vi "CIS.vi"(2 "Run uninterrupted?":bool, 3 "Device Category IN:":string(combo)="ATLAS18SS" caption="Device Category:", 4 "Batch No. IN:":string caption="Batch No.:", 5 "Wafer No. IN:":string caption="Wafer No.:", 6 "DB Serial No. IN:":string caption="DB Serial No.:") -> (0 "Done!":bool)   [LabVIEW 2018]
doc: "Performs Cis measurements according to ATLAS ITk Quality Control Specifications."
uses:
  InstrControl/Switching/Switching.lvclass
  general_VIs/globals/QC_MeasurementSetup.vi
  general_VIs/globals/QC_RunInformation.vi
  InstrControl/InstrumentSetup.vi
  InstrControl/SupplyControl/SupplyControl.lvclass
  InstrControl/LCRControl/LCRControl.lvclass
  InstrControl/ArduinoControl/ArduinoControl.lvclass
  <vilib>/Analysis/NI_AALBase.lvlib
  InstrControl/InstrControl.lvclass
panel:
  out "Tab Control 2":enum32{"Cis Setup", "Cis Scan"}(tab)
  in  "Current Limit [µA]":dbl=1000.0 min=0.0001 format="%.3f"
  in  "Cis @300V limit [pF/cm]":dbl=1.0
  in  "step interval [s] IN":i32=5 caption="step interval [s]"
  in  "step [V] IN":dbl=10.0 caption="step [V]" format="%.1f"
  in  "Final volts [V] IN":dbl=-500.0 caption="Final volts [V]"
  in  "Initial volts [V] IN":dbl caption="Initial volts [V]"
  in  "Frequency [Hz] Setup":i32=500 caption="Frequency [Hz]" format="%#.3p"
  in  "Measurement Configurations":bool
  in  "Continue":bool
  in  "Quit":bool
  in  "Software current limit?":bool
  out "Capacitance":dbl[](array[numeric]) caption="Cap [pF]"
  out "Volts":dbl[](array[numeric]) caption="Volts [V]"
  out "Resistance":dbl[](array[numeric]) caption="Res [kOhm]"
  out "step interval [s]":u32=5
  out "step [V]":dbl=10.0 format="%.1f"
  out "Final volts [V]":dbl=-700.0 format="%.1f"
  out "Initial volts [V]":dbl format="%.1f"
  out "Frequency [Hz]":i32=100000 format="%#.3p"
  out "RH":dbl[](array[numeric]) caption="RH [%]" format="%#.2f"
  out "Temp.":dbl[](array[numeric]) caption="Temp. [°C]" format="%#.2f"
  out "Cgraph":cluster{"Initial volts":dbl, dbl, dbl[]}(graph)
  in  "Scales":T1(ring)
  in  "Cscale":enum16{"1/C^2 [1/nF^2]", "nF", "pF"}(ring)=enum."pF"
  out "positive ramp?":bool
  out "Tab Control":enum32{"Cis Setup", "Cis Scan"}(tab)
  in  "LCR Meter":string(combo)="WayneKerr 6440B"
  in  "Cis Supply":string(combo)="Keithley 2410"
  in  "Temperature":enum16{"Read Arduino", "Enter manually"}(ring)
  in  "User:":string(combo)="Christoph"
  in  "Hardware Configurations":bool
  in  "Manufacturer:":string(combo)="Hamamatsu"
  in  "abort":bool
  out "Device Category:":string
  out "DB Serial No.:":string
  out "Current Volts:":dbl format="%.2f"
  in  "quit (no save)":bool
  in  "Quit & Save":bool
  out "Bias On/Off:":bool
  out "STATUS 1":string
  out "Initiated:":string
  out "Sensor No.:":string
  out "No of steps":u32
  out "Current reading No.":u32
  out "Last reading at:":string
  # "University of\nCambridge"
  # "Strip Sensor QC: inter-strip Capacitance"
  # "Vertical Scale:"
  # "Measurement Configuration"
  # "Cis Scan parameters:"
  # "Last 5 readings:"
  # "n-4"
  # "n-3"
  # "n-2"
  # "n-1"
  # "n"
  # "DUT Description"
  # "Hardware"
  # "DUT & Test Description:"
  # "Current status:"
  # "Rdg No:"
  # "out of"
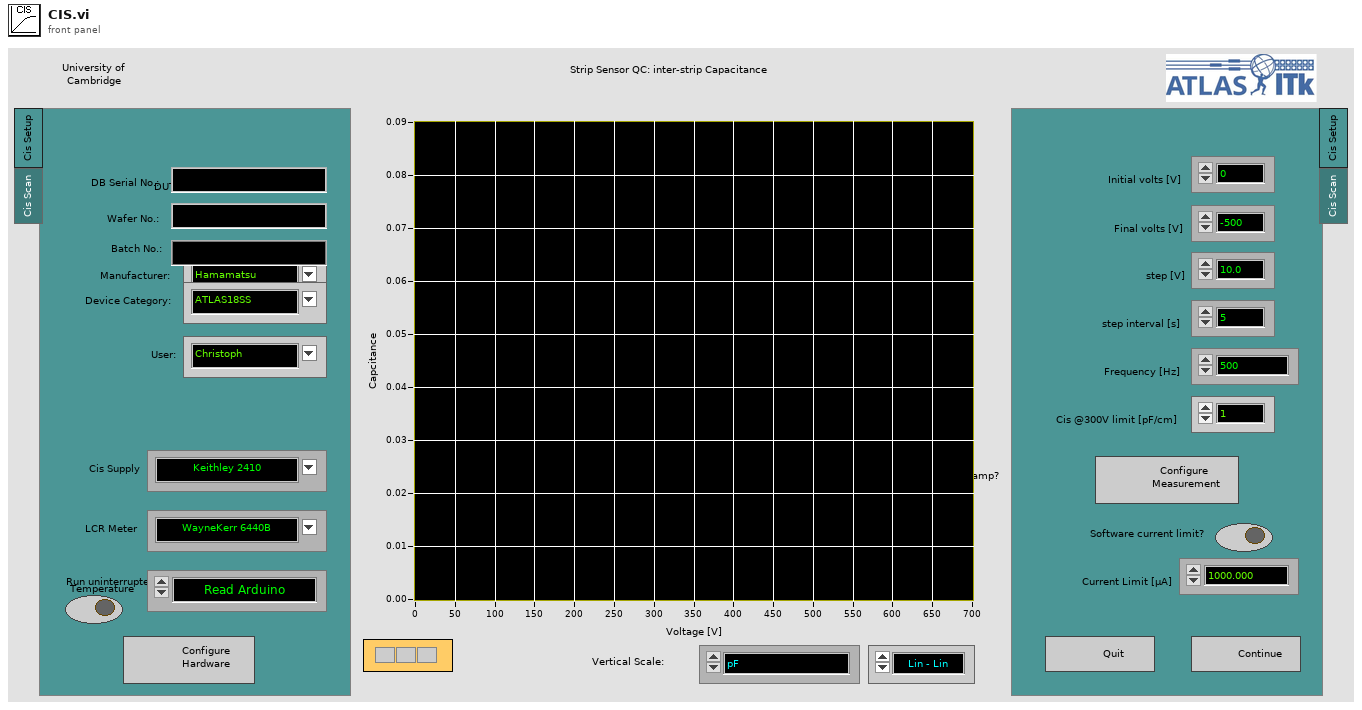
[diagram p1: front panel]
types:
  T1 = enum16{"Lin - Lin", "Log - Lin", "Lin - Log", "Log - log"}
  T2 = enum16{"Supply", "LCR", "Multimeter", "Switching"}
  T3 = enum16{"Reset", "Read Array", "Read Element", "Write Element", "Write Array", "Add Element", "Add Array"}
  T4 = enum16{"Reset", "Ground", "Striptest SMU", "Striptest LCR", "IV", "CV", "Interstrip Cap", "Interstrip Res"}
  T5 = enum32{"IV", "CV", "Stability", "Striptest", "Cis", "Ris", "PTP"}
  T6 = cluster{"Institute":string, "Manufacturers":string[], "Devices":string[], "Serialnumbers Lookup DB":string, "Data directory":string, "Backup & screenshot directory":string, "List of known users":string[], "Measurement switch not used":bool, "Measurement Switch":string, "DUT Switch":string, "Rseries IV [MOhm]":string, "Rshunt IV [MOhm]":string, "Rseries CV [MOhm]":string, "DC blocking Cap [µF]":string, "Rseries LCR [MOhm]":string, "Rseries stability [MOhm]":string, "Rshunt stability [MOhm]":string, "Rseries striptest bias [MOhm]":string, "Rseries strip pinhole [MOhm]":string}
  T7 = cluster{"Sensor Serial No.:":string, "Wafer:":string, "Batch:":string, "Manufacturer:":string, "Device Category:":string, "Database Serial No.:":string, "Date Initiated:":string, "Time Initiated:":string, "Test":string, "Probeplan used:":string, "End of Run comment:":string, "User:":string, "Vbias SMU":string, "LCR":string, "Test SMU":string, "Test DMM":string, "Comments":string, "Measurement results":cluster{"IV":string, "CV":string, "Cis":string, "Ris":string, "Stability":string, "PTP":string, "Striptest":string}}
  T8 = cluster{"Supply":refnum<class "SupplyControl.lvclass">, "LCR":refnum<class "LCRControl.lvclass">, "Arduino":refnum<class "ArduinoControl.lvclass">, "Measurement switch":refnum<class "Switching.lvclass">, "Initial Voltage [V]":dbl, "Final Voltage [V]":dbl, "Step Size [V]":dbl, "Step Interval [s]":i32, "Number Of Steps":u32, "AC frequency [Hz]":i32, "RC Configuration":u16, "AC amplitude [V]":dbl, "Ramp down steps [V]":dbl, "Ramp down Interval [s]":i32, "Set Current Limit?":bool, "Current Limit [µA]":dbl, "Temperature Readout":enum16{"Read Arduino", "Enter manually"}, "Supply Name":string, "LCR Name":string, "C_is Limit [pF/cm]":dbl, "Measurement switch used?":bool}
  T9 = cluster{"VISA address":refnum<visa-resource-name>, "T sensor":enum16{"SHT", "DS"}, "Arduino":refnum<class "ArduinoControl.lvclass">}
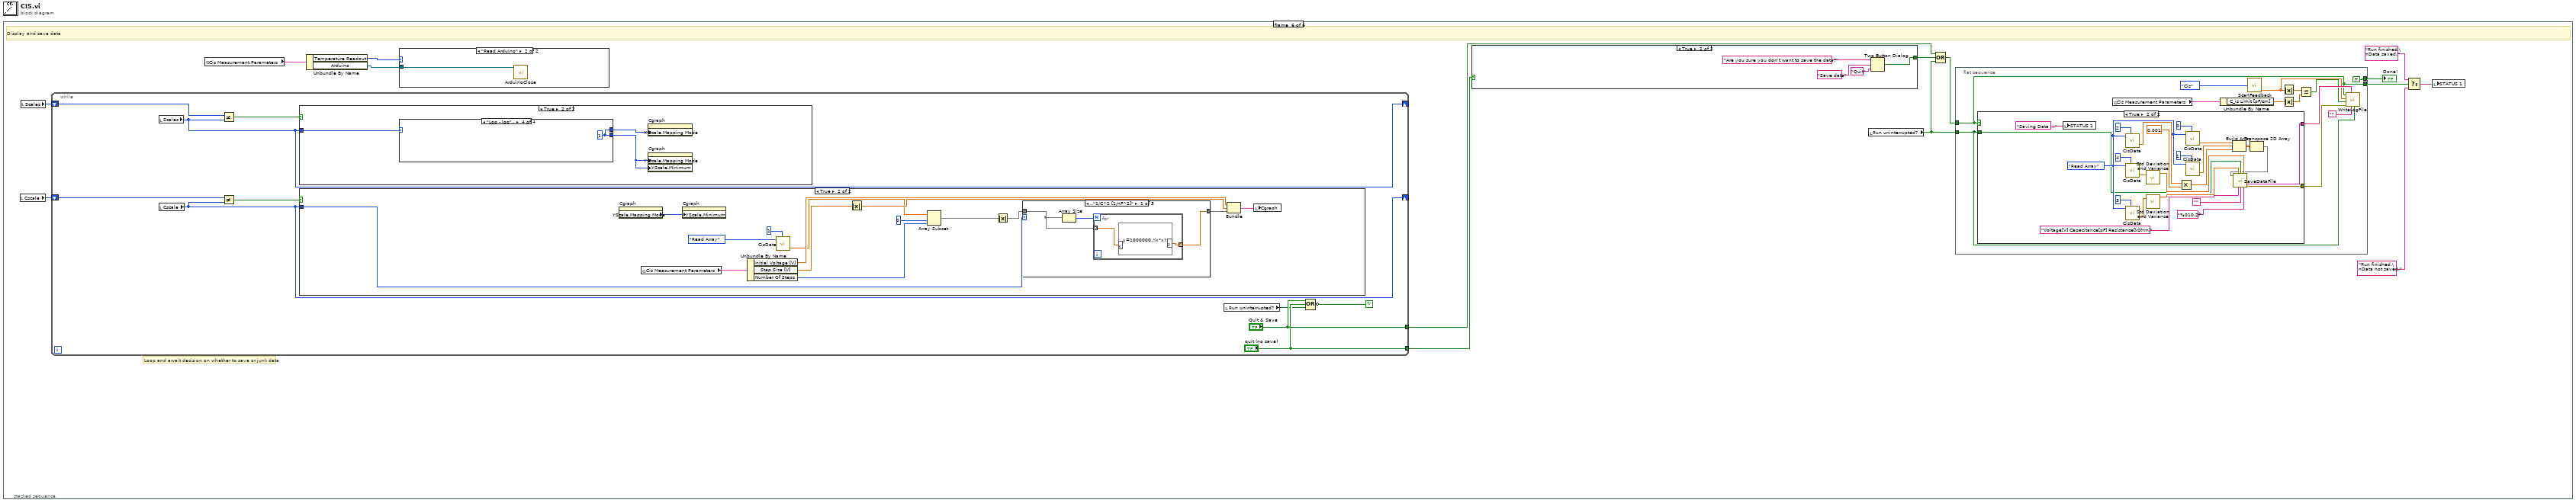
[diagram p0: block diagram]
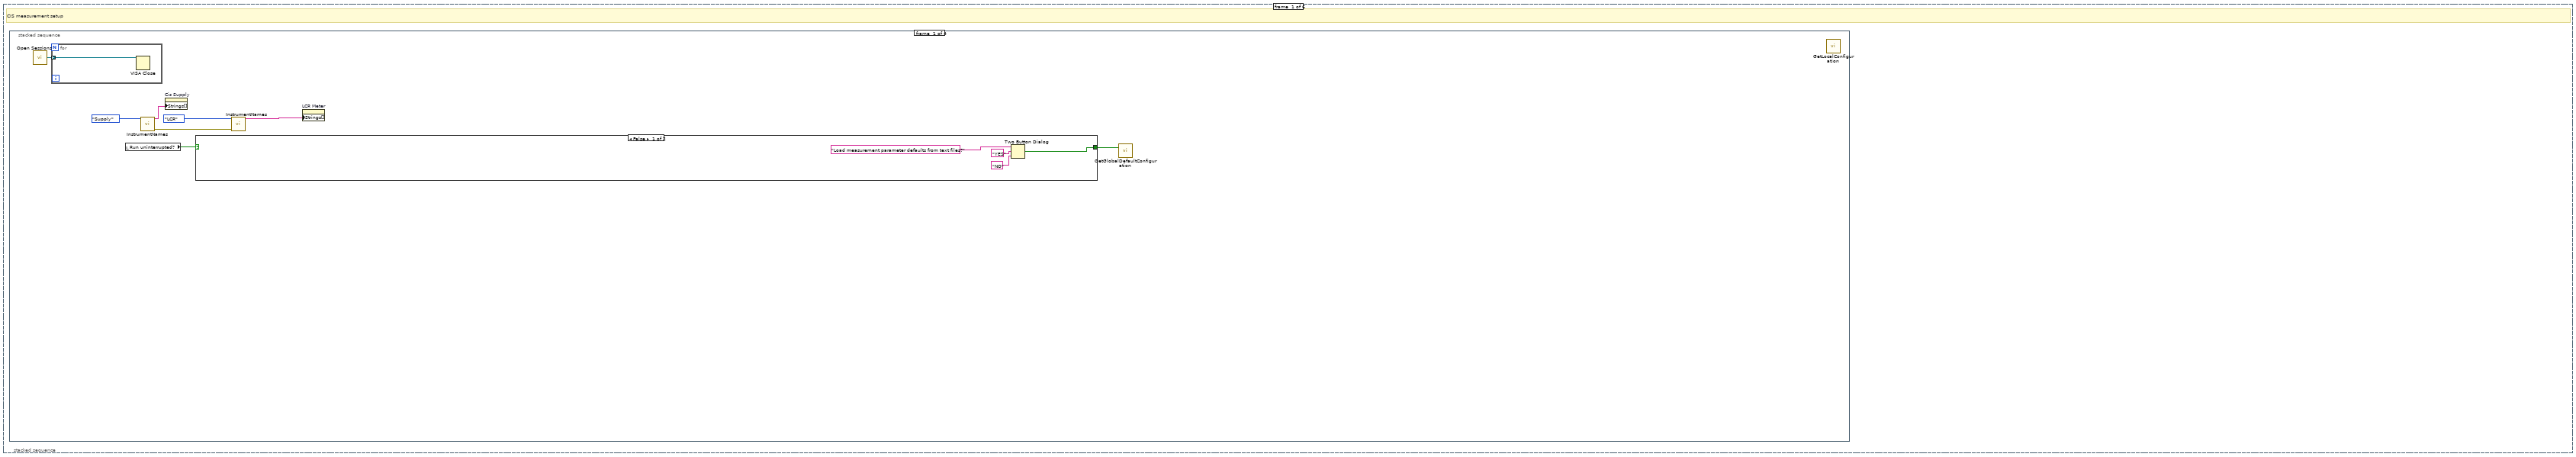
[diagram p2: hidden frame]
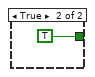
[diagram p3: hidden frame]
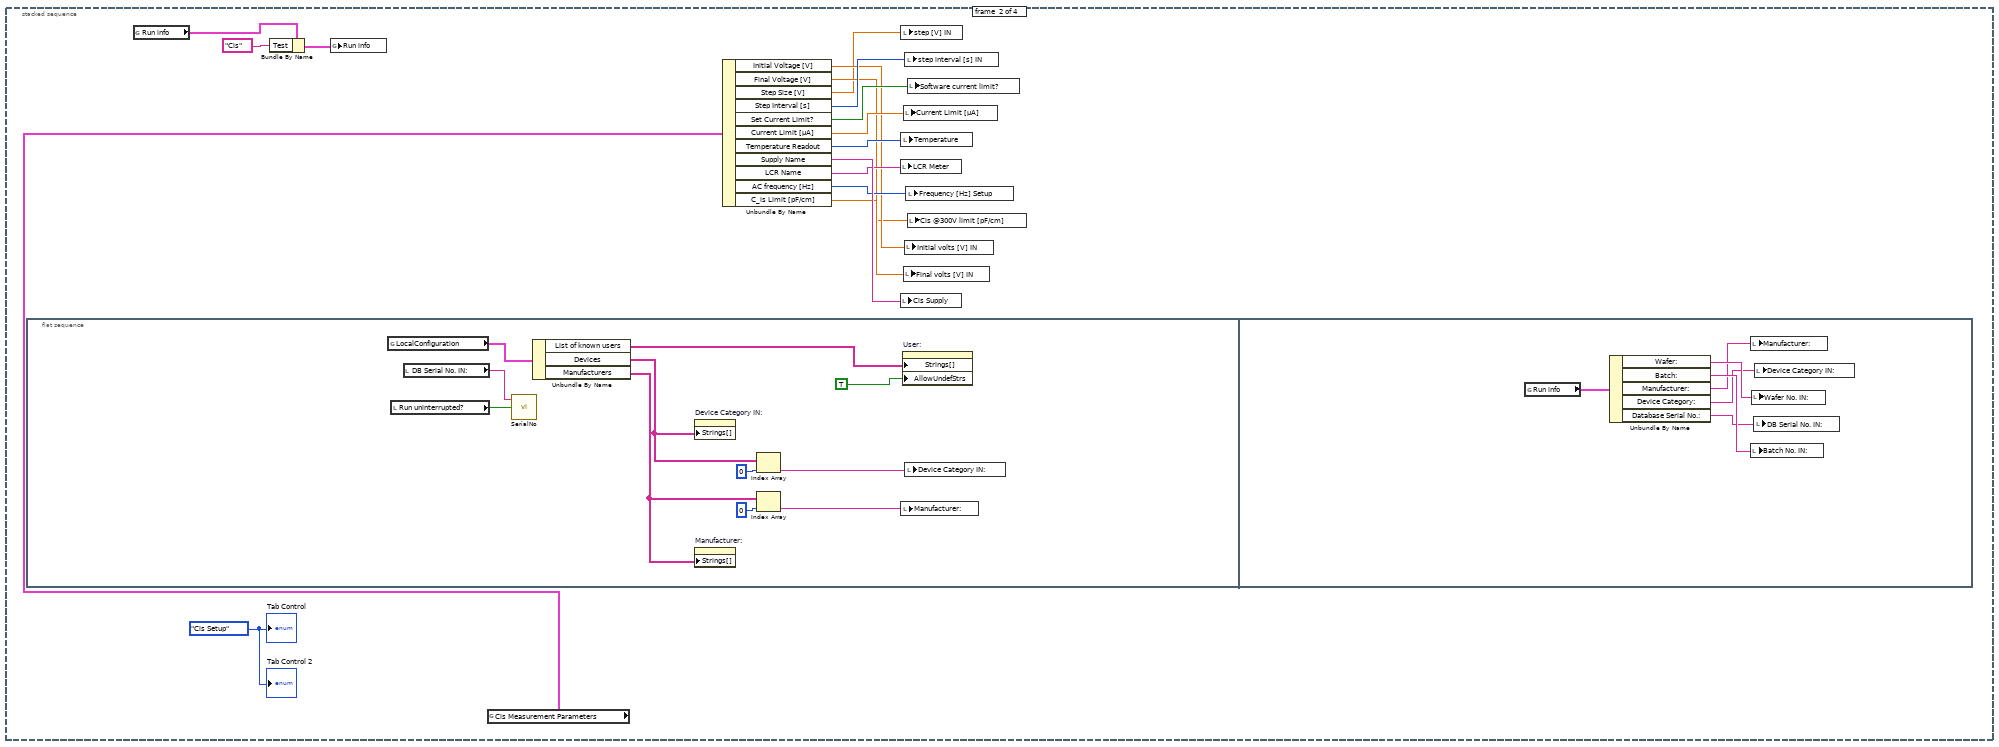
[diagram p4: hidden frame]
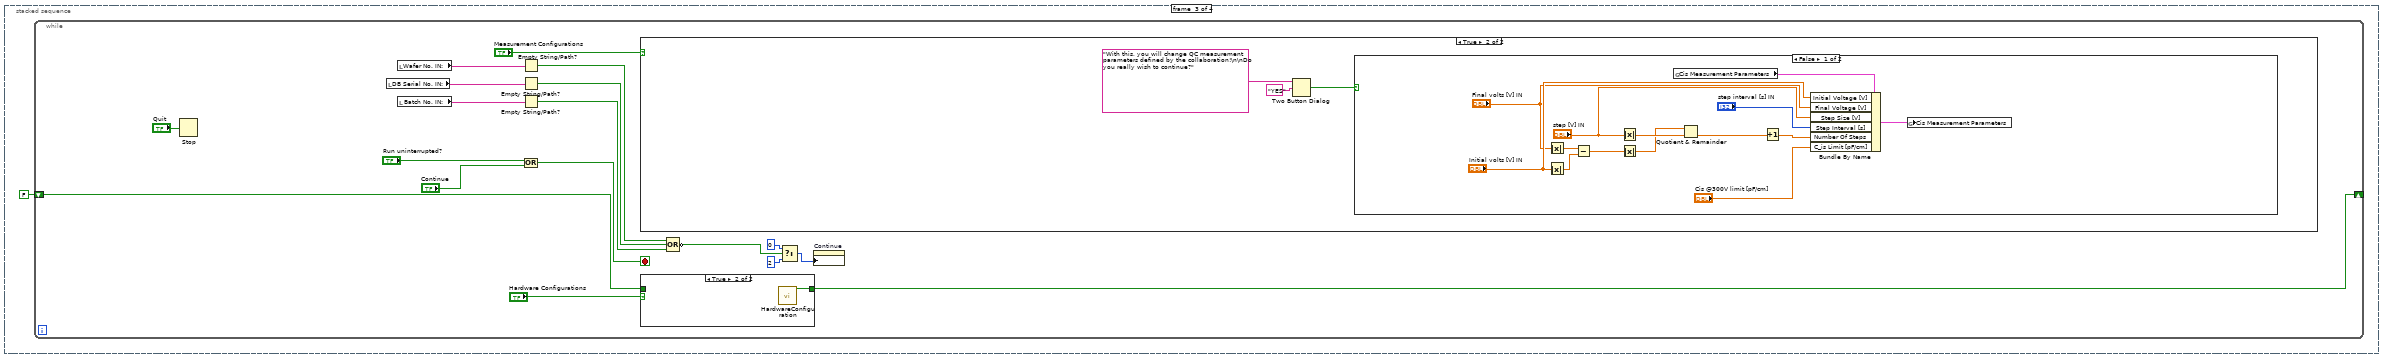
[diagram p5: hidden frame]
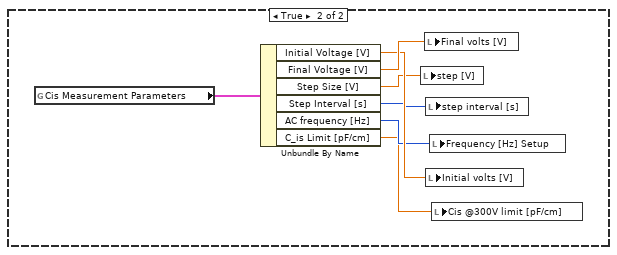
[diagram p8: hidden frame]
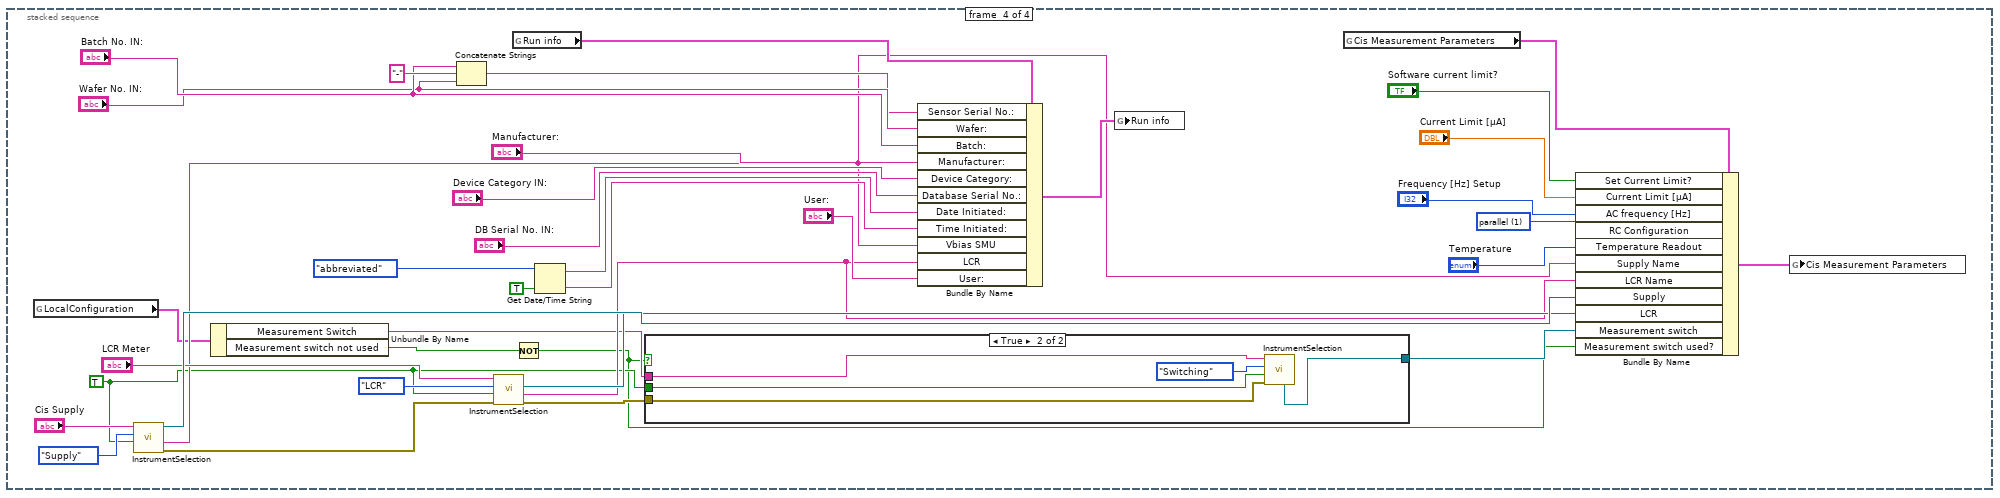
[diagram p9: hidden frame]
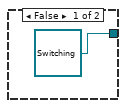
[diagram p10: hidden frame]
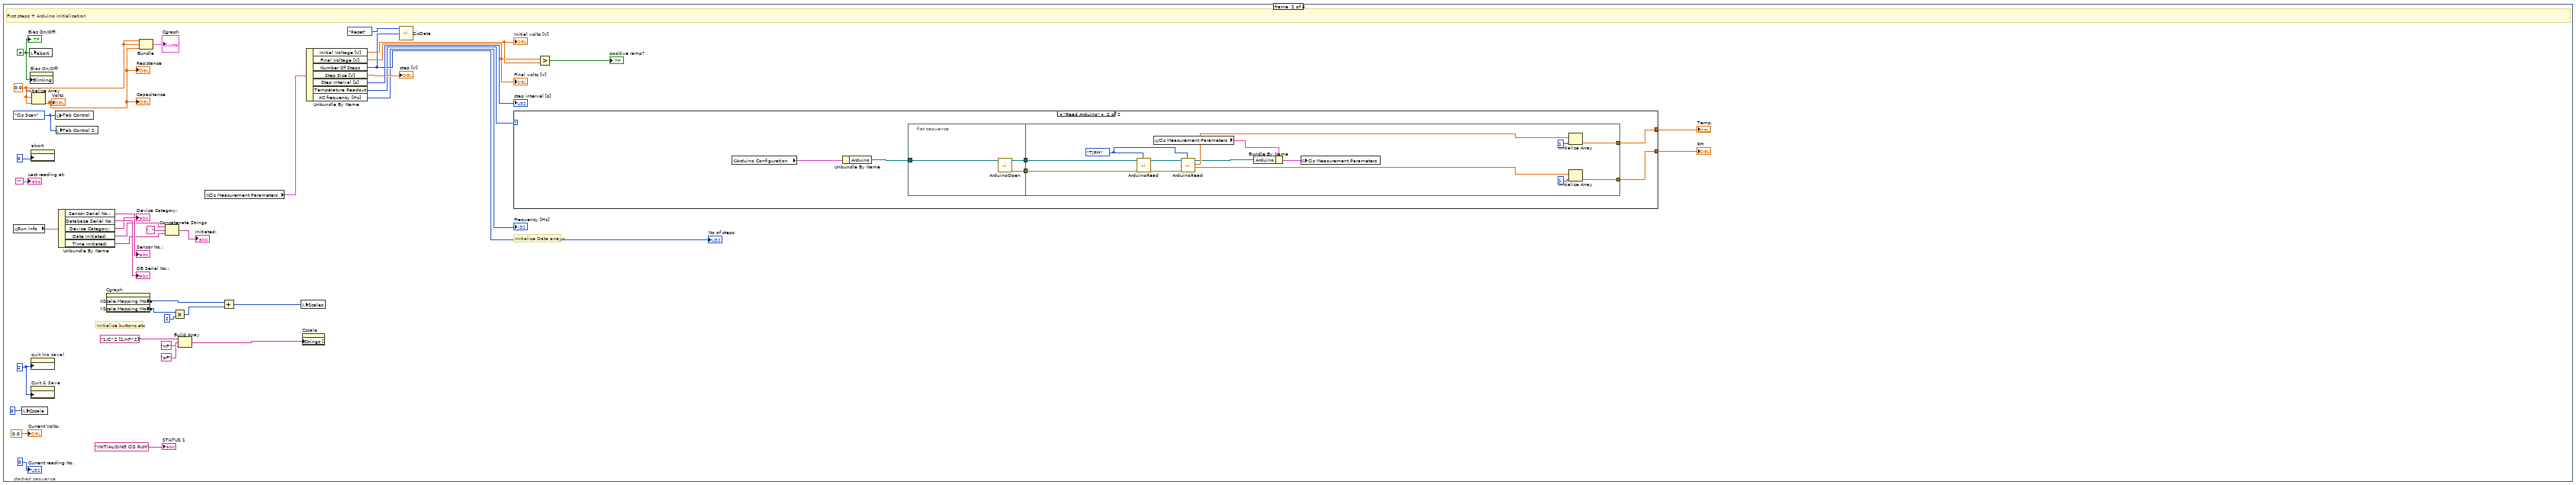
[diagram p11: hidden frame]
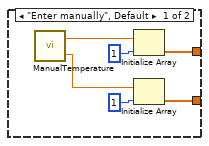
[diagram p12: hidden frame]
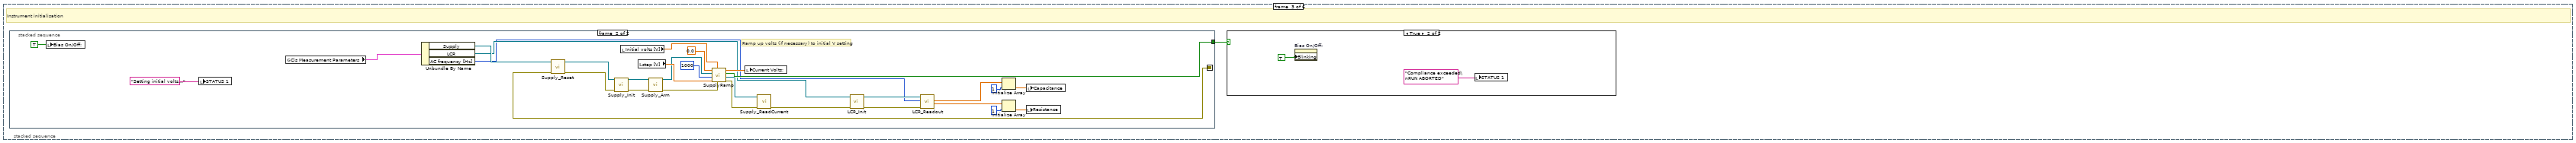
[diagram p13: hidden frame]
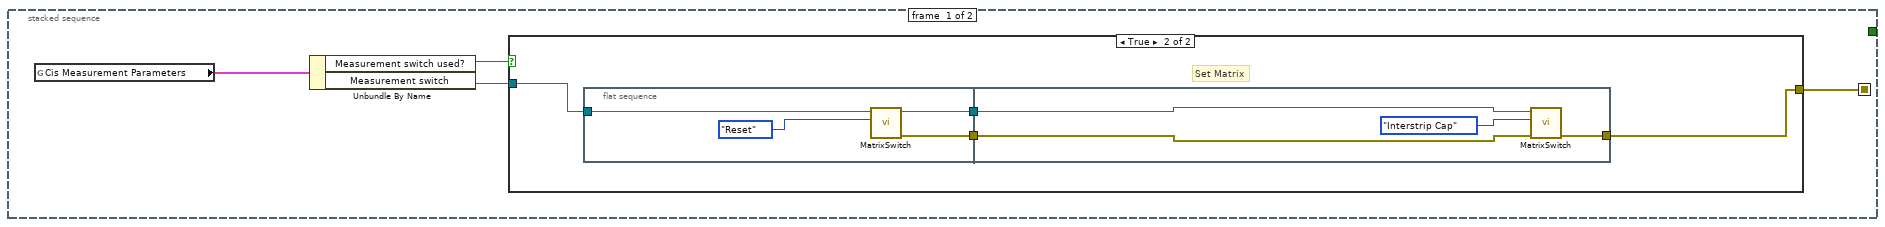
[diagram p14: hidden frame]
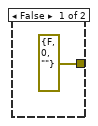
[diagram p15: hidden frame]
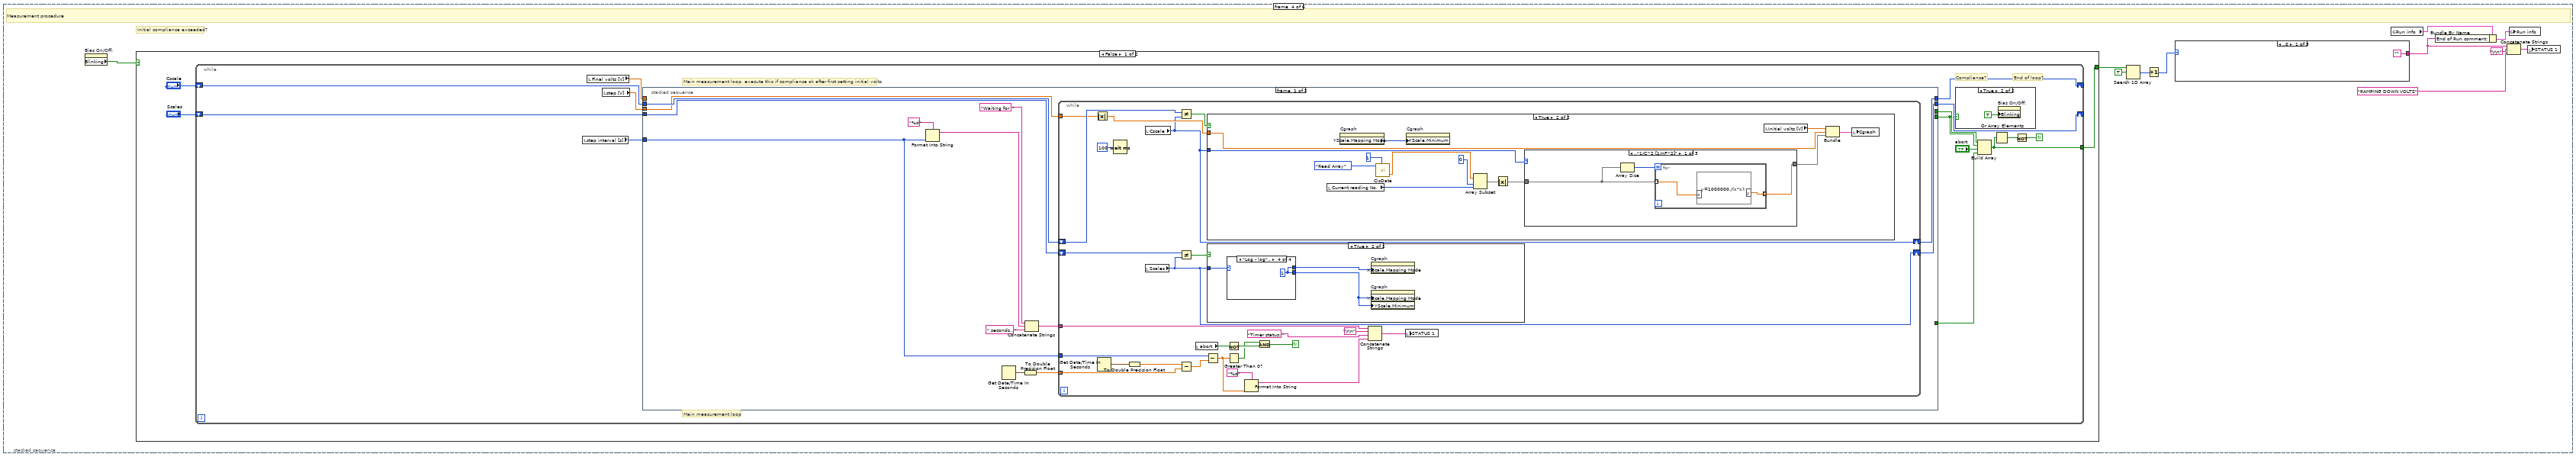
[diagram p17: hidden frame]
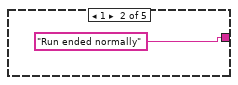
[diagram p18: hidden frame]
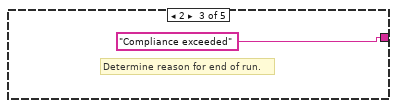
[diagram p19: hidden frame]
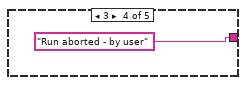
[diagram p20: hidden frame]
diagram:
  n1 = stacked-sequence {
    frame #0 {
      # "CIS measurement setup"
      n2 = stacked-sequence {
        frame #0 {
          n3 = call <vilib>:"Open Sessions.vi"() -> ("Array of Refnums"=w1:refnum<visa-resource-name>[])  [unwired: 2 in]
          n4 = for {
            tunnel: w1 -> [w9] mode=indexing
            n5 = VISA Close(VISA resource name=w9) -> ()  [unwired: 1 in, 1 out]
          }
          n6 = local read "Run uninterrupted?"() -> (w3:bool)
          n7 = call "InstrumentNames.vi"("Instrument type"=T2."Supply") -> ("error out"=w6:errorcluster, "Instrument names"=w4:string[])  [unwired: 9 in]
          n8 = property on="Cis Supply" class="CmbBox"("Strings[]"=w4) -> ()  [unwired: 2 in, 2 out]
          n9 = case shown="False" w3 {
            tunnel: [w12 TRUE] -> w2
            frame False {
              n10 = Two Button Dialog(message="Load measurement parameter defaults from text files?", 1:"NO", 2:"YES") -> (T button?=w12:bool)
            }
            frame True {
            }
          }
          n11 = call "InstrumentNames.vi"("error in (no error)"=w6, "Instrument type"=T2."LCR") -> ("Instrument names"=w5:string[])  [unwired: 8 in, 1 out]
          n12 = property on="LCR Meter" class="CmbBox"("Strings[]"=w5) -> ()  [unwired: 2 in, 2 out]
          n13 = call "GetGlobalDefaultConfiguration.vi"("Read defaults?"=w2) -> ()  [unwired: 3 in]
          n14 = call "GetLocalConfiguration.vi"() -> ()  [unwired: 3 in, 1 out]
        }
        frame #1 {
          w20 = enum32{"Cis Setup", "Cis Scan"}."Cis Setup" ("Tab Control")
          n15 = flat-sequence {
            frame #0 {
              n16 = global read "QC_RunInformation.vi" "LocalConfiguration"() -> (w37:T6)
              n17 = local read "Run uninterrupted?"() -> (w41:bool)
              n18 = local read "DB Serial No. IN:"() -> (w40:string)
              n19 = call "SerialNo.vi"("DB serial number IN"=w40, "Run uninterrupted?"=w41) -> ()  [unwired: 6 in, 2 out]
              n20 = Unbundle By Name(w37) -> ("List of known users"=w38:string[], "Devices"=w32:string[], "Manufacturers"=w35:string[])
              n21 = property on="Device Category IN:" class="CmbBox"("Strings[]"=w32) -> ()  [unwired: 2 in, 2 out]
              n22 = property on="Manufacturer:" class="CmbBox"("Strings[]"=w35) -> ()  [unwired: 2 in, 2 out]
              n23 = Index Array(array=w32, index=0) -> (element=w31:string)
              n24 = Index Array(array=w35, index=0) -> (element=w34:string)
              n25 = local write "Manufacturer:"(w34) -> ()
              n26 = property on="User:" class="CmbBox"("Strings[]"=w38, "AllowUndefStrs"=TRUE) -> ()  [unwired: 2 in, 2 out]
              n27 = local write "Device Category IN:"(w31) -> ()
            }
            frame #1 {
              n28 = global read "QC_RunInformation.vi" "Run info"() -> (w42:T7)
              n29 = Unbundle By Name(w42) -> ("Wafer:"=w47:string, "Batch:"=w46:string, "Manufacturer:"=w45:string, "Device Category:"=w43:string, "Database Serial No.:"=w44:string)
              n30 = local write "Manufacturer:"(w45) -> ()
              n31 = local write "Batch No. IN:"(w46) -> ()
              n32 = local write "Wafer No. IN:"(w47) -> ()
              n33 = local write "DB Serial No. IN:"(w44) -> ()
              n34 = local write "Device Category IN:"(w43) -> ()
            }
          }
          n35 = global read "QC_RunInformation.vi" "Run info"() -> (w21:T7)
          n36 = Bundle By Name(cluster=w21, "Test"="Cis") -> (w23:T7)
          n37 = global write "QC_RunInformation.vi" "Run info"(w23) -> ()
          n38 = global read "QC_MeasurementSetup.vi" "Cis Measurement Parameters"() -> (w28:T8)
          n39 = Unbundle By Name(w28) -> ("Initial Voltage [V]"=w17:dbl, "Final Voltage [V]"=w18:dbl, "Step Size [V]"=w16:dbl, "Step Interval [s]"=w19:i32, "Set Current Limit?"=w27:bool, "Current Limit [µA]"=w26:dbl, "Temperature Readout"=w30:enum16{"Read Arduino", "Enter manually"}, "Supply Name"=w29:string, "LCR Name"=w25:string, "AC frequency [Hz]"=w24:i32, "C_is Limit [pF/cm]"=w15:dbl)
          n40 = local write "LCR Meter"(w25) -> ()
          n41 = local write "Cis Supply"(w29) -> ()
          n42 = local write "step [V] IN"(w16) -> ()
          n43 = local write "Temperature"(w30) -> ()
          n44 = local write "Current Limit [µA]"(w26) -> ()
          n45 = local write "Final volts [V] IN"(w18) -> ()
          n46 = local write "Initial volts [V] IN"(w17) -> ()
          n47 = local write "step interval [s] IN"(w19) -> ()
          n48 = local write "Frequency [Hz] Setup"(w24) -> ()
          n49 = local write "Software current limit?"(w27) -> ()
          n50 = local write "Cis @300V limit [pF/cm]"(w15) -> ()
          "Tab Control" <- w20
          "Tab Control 2" <- w20
        }
        frame #2 {
          n51 = while {
            shift-right: [w49] -> _
            shift-left: FALSE -> [w50]
            stop <- w53 stop-if-true
            n52 = Stop(stop? (T)="Quit") -> ()
            n53 = local read "DB Serial No. IN:"() -> (w64:string)
            n54 = local read "Wafer No. IN:"() -> (w65:string)
            n55 = local read "Batch No. IN:"() -> (w57:string)
            n56 = Empty String/Path?(string/path=w65) -> (empty?=w62:bool)
            n57 = Empty String/Path?(string/path=w64) -> (empty?=w63:bool)
            n58 = Empty String/Path?(string/path=w57) -> (empty?=w56:bool)
            n59 = Or(x="Run uninterrupted?", y="Continue") -> (x .or. y?=w53:bool)
            n60 = case shown="True" "Measurement Configurations" {
              frame False {
              }
              frame True {
                n61 = Two Button Dialog(message="With this, you will change QC measurement parameters defined by the collaboration!\n\nDo you really wish to continue?", 2:"YES") -> (T button?=w69:bool)  [unwired: 1 in]
                n62 = case shown="False" w69 {
                  frame False {
                    n63 = Absolute Value(x="Final volts [V] IN") -> (abs(x)=w82:dbl)
                    n64 = Absolute Value(x="Initial volts [V] IN") -> (abs(x)=w81:dbl)
                    n65 = Subtract(x=w82, y=w81) -> (x-y=w79:dbl)
                    n66 = Absolute Value(x="step [V] IN") -> (abs(x)=w80:dbl)
                    n67 = Absolute Value(x=w79) -> (abs(x)=w75:dbl)
                    n68 = global read "QC_MeasurementSetup.vi" "Cis Measurement Parameters"() -> (w84:T8)
                    n69 = Quotient & Remainder(x=w75, y=w80) -> (floor(x/y)=w83:dbl)  [unwired: 1 out]
                    n70 = Increment(x=w83) -> (x+1=w78:dbl)
                    n71 = Bundle By Name(cluster=w84, "Initial Voltage [V]"="Initial volts [V] IN", "Final Voltage [V]"="Final volts [V] IN", "Step Size [V]"="step [V] IN", "Step Interval [s]"="step interval [s] IN", "Number Of Steps"=w78, "C_is Limit [pF/cm]"="Cis @300V limit [pF/cm]") -> (w85:T8)
                    n72 = global write "QC_MeasurementSetup.vi" "Cis Measurement Parameters"(w85) -> ()
                  }
                  frame True {
                    n73 = global read "QC_MeasurementSetup.vi" "Cis Measurement Parameters"() -> (w92:T8)
                    n74 = Unbundle By Name(w92) -> ("Initial Voltage [V]"=w90:dbl, "Final Voltage [V]"=w91:dbl, "Step Size [V]"=w89:dbl, "Step Interval [s]"=w88:i32, "AC frequency [Hz]"=w87:i32, "C_is Limit [pF/cm]"=w86:dbl)
                    n75 = local write "step [V]"(w89) -> ()
                    n76 = local write "Final volts [V]"(w91) -> ()
                    n77 = local write "step interval [s]"(w88) -> ()
                    n78 = local write "Initial volts [V]"(w90) -> ()
                    n79 = local write "Frequency [Hz] Setup"(w87) -> ()
                    n80 = local write "Cis @300V limit [pF/cm]"(w86) -> ()
                  }
                }
              }
            }
            n81 = case shown="True" "Hardware Configurations" {
              tunnel: [w67 w68] -> w49
              tunnel: w50 -> [w67 _]
              frame False {
              }
              frame True {
                n82 = call "HardwareConfiguration.vi"() -> ("configured?"=w68:bool)  [unwired: 11 in]
              }
            }
            n83 = Compound Arithmetic op=OR(w62, w63, w56) -> (invert w61:bool)
            n84 = Select(t=0, s=w61, f=2) -> (s? t:f=w58:i32)
            n85 = property on="Continue" class="Bool"("DisabledEnum"=w58) -> ()  [unwired: 2 in, 2 out]
          }
        }
        frame #3 {
          w98 = TRUE
          w118 = u16 1 items=["serial", "parallel"] ("RC Configuration")
          n86 = global read "QC_RunInformation.vi" "LocalConfiguration"() -> (w96:T6)
          n87 = call "InstrumentSelection.vi"("Verify GPIB address"=w98, "Instrument type"=T2."Supply", "Instrument name IN"="Cis Supply") -> ("error out"=w112:errorcluster, "Instrument name OUT"=w101:string, "Supply"=w115:refnum<class "SupplyControl.lvclass">)  [unwired: 3 in, 3 out]
          n88 = Unbundle By Name(w96) -> ("Measurement Switch"=w95:string, "Measurement switch not used"=w94:bool)
          n89 = Concatenate Strings("Batch No. IN:", "-", "Wafer No. IN:") -> (w102:string)
          n90 = call "InstrumentSelection.vi"("error in (no error)"=w112, "Verify GPIB address"=w98, "Instrument type"=T2."LCR", "Instrument name IN"="LCR Meter") -> ("error out"=w99:errorcluster, "Instrument name OUT"=w100:string, "LCR"=w114:refnum<class "LCRControl.lvclass">)  [unwired: 2 in, 3 out]
          n91 = global read "QC_RunInformation.vi" "Run info"() -> (w123:T7)
          n92 = Not(x=w94) -> (.not. x?=w93:bool)
          n93 = Get Date/Time String(date format (0)=enum16{"short", "long", "abbreviated"}."abbreviated", want seconds? (F)=TRUE) -> (date string=w107:string, time string=w106:string)  [unwired: 1 in]
          n94 = case shown="True" w93 {
            tunnel: w99 -> [_ w134]
            tunnel: [refnum<class "Switching.lvclass"> refnum ("Switching") w133] -> w97
            tunnel: w98 -> [_ w132]
            tunnel: w95 -> [_ w131]
            frame False {
            }
            frame True {
              n95 = call "InstrumentSelection.vi"("error in (no error)"=w134, "Verify GPIB address"=w132, "Instrument type"=T2."Switching", "Instrument name IN"=w131) -> ("Switching"=w133:refnum<class "Switching.lvclass">)  [unwired: 2 in, 5 out]
            }
          }
          n96 = Bundle By Name(cluster=w123, "Sensor Serial No.:"=w102, "Wafer:"="Wafer No. IN:", "Batch:"="Batch No. IN:", "Manufacturer:"="Manufacturer:", "Device Category:"="Device Category IN:", "Database Serial No.:"="DB Serial No. IN:", "Date Initiated:"=w107, "Time Initiated:"=w106, "Vbias SMU"=w101, "LCR"=w100, "User:"="User:") -> (w122:T7)
          n97 = global write "QC_RunInformation.vi" "Run info"(w122) -> ()
          n98 = global read "QC_MeasurementSetup.vi" "Cis Measurement Parameters"() -> (w128:T8)
          n99 = Bundle By Name(cluster=w128, "Set Current Limit?"="Software current limit?", "Current Limit [µA]"="Current Limit [µA]", "AC frequency [Hz]"="Frequency [Hz] Setup", "RC Configuration"=w118, "Temperature Readout"="Temperature", "Supply Name"=w101, "LCR Name"=w100, "Supply"=w115, "LCR"=w114, "Measurement switch"=w97, "Measurement switch used?"=w93) -> (w129:T8)
          n100 = global write "QC_MeasurementSetup.vi" "Cis Measurement Parameters"(w129) -> ()
        }
      }
    }
    frame #1 {
      w141 = enum32{"Cis Setup", "Cis Scan"}."Cis Scan" ("Tab Control")
      w158 = 2
      w165 = 0.0
      w157 = FALSE ("Visible")
      # "Initialise buttons etc"
      # "Initialise Data arrays"
      # "First steps + Arduino initialisation"
      n101 = global read "QC_RunInformation.vi" "Run info"() -> (w175:T7)
      n102 = local write "Cscale"(u16 0 ("Scale")) -> ()
      n103 = local write "abort"(w157) -> ()
      n104 = property on="Bias On/Off:" class="Bool (strict)"("Blinking"=w157) -> ()  [unwired: 2 in, 2 out]
      n105 = property on="abort" class="Bool (strict)"("DisabledEnum"=0) -> ()  [unwired: 2 in, 2 out]
      n106 = property on="quit (no save)" class="Bool"("DisabledEnum"=w158) -> ()  [unwired: 2 in, 2 out]
      n107 = property on="Quit & Save" class="Bool"("DisabledEnum"=w158) -> ()  [unwired: 2 in, 2 out]
      n108 = Initialize Array(w165, w165) -> (w143:dbl[])
      "Volts" <- w143
      "Capacitance" <- w143
      "Resistance" <- w143
      n109 = local write "Tab Control"(w141) -> ()
      n110 = local write "Tab Control 2"(w141) -> ()
      n111 = Unbundle By Name(w175) -> ("Sensor Serial No.:"=→"Sensor No.:":string, "Database Serial No.:"=→"DB Serial No.:":string, "Device Category:"=→"Device Category:":string, "Date Initiated:"=w138:string, "Time Initiated:"=w137:string)
      n112 = property on="Cgraph" class="WFGraph (strict)"() -> ("XScale.Mapping Mode"=w150:u8, "YScale.Mapping Mode"=w149:u8)  [unwired: 2 in, 2 out]
      n113 = Bundle(w165, w165, w143) -> (→"Cgraph":cluster{dbl, dbl, dbl[]})  [unwired: 1 in]
      n114 = Concatenate Strings(w138, ", ", w137) -> (→"Initiated:":string)
      n115 = Multiply(x=w149, y=2) -> (x*y=w152:i32)
      n116 = Build Array("1/C^2 [1/nF^2]", "nF", "pF") -> (w172:string[])
      n117 = global read "QC_MeasurementSetup.vi" "Cis Measurement Parameters"() -> (w146:T8)
      n118 = Add(x=w150, y=w152) -> (x+y=w148:i32)
      n119 = local write "Scales"(w148) -> ()
      n120 = property on="Cscale" class="Enum (strict)"("Strings []"=w172) -> ()  [unwired: 2 in, 2 out]
      n121 = Unbundle By Name(w146) -> ("Initial Voltage [V]"=w156:dbl, "Final Voltage [V]"=w155:dbl, "Number Of Steps"=w166:u32, "Step Size [V]"=→"step [V]":dbl, "Step Interval [s]"=→"step interval [s]":i32, "Temperature Readout"=w159:enum16{"Read Arduino", "Enter manually"}, "AC frequency [Hz]"=→"Frequency [Hz]":i32)
      "No of steps" <- w166
      "Initial volts [V]" <- w156
      "Final volts [V]" <- w155
      n122 = call "CisData.vi"("Action"=T3."Reset", "Array Size / Index"=w166) -> ()  [unwired: 3 in, 2 out]
      n123 = case shown="\"Read Arduino\"" w159 {
        tunnel: [w181 w188] -> w162
        tunnel: [w178 w187] -> w147
        frame "Enter manually", Default {
          n124 = call "ManualTemperature.vi"() -> ("Humidity [%] out"=w177:dbl, "Temperature [°C] out"=w182:dbl)
          n125 = Initialize Array(w182, 1) -> (w181:dbl[])
          n126 = Initialize Array(w177, 1) -> (w178:dbl[])
        }
        frame "Read Arduino" {
          n127 = global read "InstrumentSetup.vi" "Arduino Configuration"() -> (w184:T9)
          n128 = Unbundle By Name(w184) -> ("Arduino"=w183:refnum<class "ArduinoControl.lvclass">)
          n129 = flat-sequence {
            tunnel: [w189] -> w186
            tunnel: [w191] -> w185
            tunnel: w183 -> [w190]
            tunnel: [w205] -> w188
            tunnel: [w202] -> w187
            tunnel: w186 -> [w194]
            tunnel: w185 -> [w195]
            frame #0 {
              n130 = call "ArduinoOpen.vi"("ArduinoControl in"=w190) -> ("error out"=w191:errorcluster, "ArduinoControl out"=w189:refnum<class "ArduinoControl.lvclass">)  [unwired: 9 in]
            }
            frame #1 {
              w196 = enum16{"T/RH", "Interlock", "Edgesense"}."T/RH" ("Arduino function")
              n131 = call "ArduinoRead.vi"("Arduino function"=w196, "error in (no error)"=w195, "ArduinoControl in"=w194) -> ("error out"=w192:errorcluster, "ArduinoControl out"=w193:refnum<class "ArduinoControl.lvclass">)  [unwired: 3 in, 4 out]
              n132 = global read "QC_MeasurementSetup.vi" "Cis Measurement Parameters"() -> (w198:T8)
              n133 = call "ArduinoRead.vi"("Arduino function"=w196, "error in (no error)"=w192, "ArduinoControl in"=w193) -> ("rel. Humidity [%]"=w200:dbl, "Temperature [°C]"=w201:dbl, "ArduinoControl out"=w199:refnum<class "ArduinoControl.lvclass">)  [unwired: 3 in, 3 out]
              n134 = Bundle By Name(cluster=w198, "Arduino"=w199) -> (w197:T8)
              n135 = global write "QC_MeasurementSetup.vi" "Cis Measurement Parameters"(w197) -> ()
              n136 = Initialize Array(w201, 1) -> (w205:dbl[])
              n137 = Initialize Array(w200, 1) -> (w202:dbl[])
            }
          }
        }
      }
      "Temp." <- w162
      "RH" <- w147
      n138 = Greater?(x=w155, y=w156) -> (0:→"positive ramp?":bool)
      "STATUS 1" <- "INITIALISING CIS RUN"
      "Bias On/Off:" <- w157
      "Last reading at:" <- ""
      "Current reading No." <- u32 0 ("Current reading No.")
      "Current Volts:" <- 0.0 ("Current Volts:")
    }
    frame #2 {
      # "Instrument initialisation"
      n139 = stacked-sequence {
        seq-local: [w208 _] -> [_ w227]
        tunnel: [_ w228] -> w206
        frame #0 {
          n140 = global read "QC_MeasurementSetup.vi" "Cis Measurement Parameters"() -> (w207:T8)
          n141 = Unbundle By Name(w207) -> ("Measurement switch used?"=w210:bool, "Measurement switch"=w209:refnum<class "Switching.lvclass">)
          n142 = case shown="True" w210 {
            tunnel: w209 -> [_ w212]
            tunnel: [errorcluster {"status"=FALSE, "code"=0, "source"=""} ("error constant") w213] -> w208
            frame False {
            }
            frame True {
              # "Set Matrix"
              n143 = flat-sequence {
                tunnel: [w219] -> w215
                tunnel: [w218] -> w214
                tunnel: w212 -> [w216]
                tunnel: w215 -> [w223]
                tunnel: w214 -> [w222]
                tunnel: [w221] -> w213
                frame #0 {
                  n144 = call-dynamic "MatrixSwitch.vi"("Action"=T4."Reset", "Switching in"=w216) -> ("error out"=w219:errorcluster, "Switching out"=w218:refnum<class "Switching.lvclass">)  [unwired: 7 in, 1 out]
                }
                frame #1 {
                  n145 = call-dynamic "MatrixSwitch.vi"("error in (no error)"=w223, "Action"=T4."Interstrip Cap", "Switching in"=w222) -> ("error out"=w221:errorcluster)  [unwired: 6 in, 2 out]
                }
              }
            }
          }
        }
        frame #1 {
          # "Ramp up volts (if necessary) to initial V setting"
          n146 = local write "Bias On/Off:"(TRUE ("Compliance?")) -> ()
          n147 = local write "STATUS 1"("Setting initial volts..." ("STATUS 1")) -> ()
          n148 = global read "QC_MeasurementSetup.vi" "Cis Measurement Parameters"() -> (w249:T8)
          n149 = Unbundle By Name(w249) -> ("Supply"=w246:refnum<class "SupplyControl.lvclass">, "LCR"=w225:refnum<class "LCRControl.lvclass">, "AC frequency [Hz]"=w224:i32)
          n150 = call-dynamic "Supply_Reset.vi"("error in (no error)"=w227, "SupplyControl in"=w246) -> ("error out"=w251:errorcluster, "SupplyControl out"=w253:refnum<class "SupplyControl.lvclass">)  [unwired: 8 in]
          n151 = call-dynamic "Supply_Init.vi"("error in (no error)"=w251, "SupplyControl in"=w253) -> ("error out"=w250:errorcluster, "SupplyControl out"=w252:refnum<class "SupplyControl.lvclass">)  [unwired: 8 in]
          n152 = local read "Initial volts [V]"() -> (w231:dbl)
          n153 = local read "step [V]"() -> (w232:dbl)
          n154 = call-dynamic "Supply_Arm.vi"("error in (no error)"=w250, "SupplyControl in"=w252) -> ("error out"=w229:errorcluster, "SupplyControl out"=w230:refnum<class "SupplyControl.lvclass">)  [unwired: 8 in]
          n155 = call "SupplyRamp.vi"("error in"=w229, "Requested Voltage"=w231, "Step Size"=w232, "Step Delay"=1000, "Supply IN"=w230, "Starting Voltage"=0.0) -> ("error out"=w245:errorcluster, "Supply OUT"=w226:refnum<class "SupplyControl.lvclass">, "Compliance exceeded"=w228:bool, "Current Voltage"=w235:dbl)  [unwired: 2 in]
          n156 = local write "Current Volts:"(w235) -> ()
          n157 = call-dynamic "Supply_ReadCurrent.vi"("error in (no error)"=w245, "SupplyControl in"=w226) -> ("error out"=w242:errorcluster)  [unwired: 7 in, 2 out]
          n158 = call-dynamic "LCR_Init.vi"("error in (no error)"=w242, "LCRControl in"=w225) -> ("error out"=w244:errorcluster, "LCRControl out"=w243:refnum<class "LCRControl.lvclass">)  [unwired: 8 in]
          n159 = call-dynamic "LCR_Readout.vi"("error in (no error)"=w244, "Frequency in Hz"=w224, "LCRControl in"=w243) -> ("Resistance in Ohm"=w240:dbl, "Capacitance in pF"=w241:dbl)  [unwired: 5 in, 2 out]
          n160 = Initialize Array(w241, 1) -> (w236:dbl[])
          n161 = Initialize Array(w240, 1) -> (w239:dbl[])
          n162 = local write "Resistance"(w239) -> ()
          n163 = local write "Capacitance"(w236) -> ()
        }
      }
      n164 = case shown="True" w206 {
        frame False {
        }
        frame True {
          n165 = property on="Bias On/Off:" class="Bool (strict)"("Blinking"=TRUE) -> ()  [unwired: 2 in, 2 out]
          n166 = local write "STATUS 1"("Compliance exceeded\nRUN ABORTED") -> ()
        }
      }
    }
    frame #3 {
      # "Initial compliance exceeded?"
      # "Measurement procedure"
      n167 = property on="Bias On/Off:" class="Bool (strict)"() -> ("Blinking"=w266:bool)  [unwired: 2 in, 2 out]
      n168 = case shown="False" w266 {
        tunnel: [w274 w521] -> w265
        frame False {
          n169 = while {
            shift-left: "Cscale" -> [w284]
            shift-right: [w283] -> _
            shift-left: "Scales" -> [w285]
            shift-right: [w286] -> _
            tunnel: [w282] -> w274
            stop <- w287 continue-if-true
            # "Main measurement loop"
            # "End of loop?"
            # "Compliance?"
            # "Main measurement loop. execute this if compliance ok after first setting initial volts"
            n170 = local read "step interval [s]"() -> (w279:u32)
            n171 = local read "Final volts [V]"() -> (w280:dbl)
            n172 = local read "step [V]"() -> (w281:dbl)
            n173 = stacked-sequence {
              tunnel: [w301 _] -> w286
              tunnel: w281 -> [w298 w364]
              tunnel: [_ w363] -> w276
              tunnel: w280 -> [_ w362]
              tunnel: w279 -> [w289 w361]
              tunnel: [_ w360] -> w278
              tunnel: w285 -> [w300 _]
              tunnel: w284 -> [w299 _]
              tunnel: [w297 _] -> w283
              tunnel: [_ w358] -> w277
              frame #0 {
                n174 = Format Into String(format string="%d", w289) -> (resulting string=w294:string)  [unwired: 2 in, 1 out]
                n175 = Get Date/Time In Seconds() -> (seconds since 1Jan1904=w291:timestamp)
                n176 = To Double Precision Float(number=w291) -> (double precision float=w292:dbl)
                n177 = Concatenate Strings("Waiting for  ", w294, " seconds...") -> (w290:string)
                n178 = while {
                  tunnel: w298 -> [w310]
                  shift-left: w299 -> [w314]
                  shift-right: [w307] -> w297
                  shift-left: w300 -> [w315]
                  shift-right: [w316] -> w301
                  tunnel: w290 -> [w308]
                  tunnel: w289 -> [w320]
                  tunnel: w292 -> [w321]
                  stop <- w322 continue-if-true
                  n179 = Absolute Value(x=w310) -> (abs(x)=w309:dbl)
                  n180 = Get Date/Time In Seconds() -> (seconds since 1Jan1904=w306:timestamp)
                  n181 = Wait (ms)(milliseconds to wait=u32 100) -> ()  [unwired: 1 out]
                  n182 = To Double Precision Float(number=w306) -> (double precision float=w326:dbl)
                  n183 = local read "Cscale"() -> (w307:enum16{"1/C^2 [1/nF^2]", "nF", "pF"})
                  n184 = local read "Scales"() -> (w316:T1)
                  n185 = Not Equal?(x=w314, y=w307) -> (x != y?=w305:bool)
                  n186 = Not Equal?(x=w315, y=w316) -> (x != y?=w317:bool)
                  n187 = Subtract(x=w326, y=w321) -> (x-y=w303:dbl)
                  n188 = local read "abort"() -> (w319:bool)
                  n189 = Subtract(x=w320, y=w303) -> (x-y=w302:dbl)
                  n190 = case shown="True" w305 {
                    tunnel: w309 -> [_ w338]
                    tunnel: w307 -> [_ w331]
                    frame False {
                    }
                    frame True {
                      n191 = local read "Current reading No."() -> (w336:u32)
                      n192 = property on="Cgraph" class="WFGraph (strict)"() -> ("YScale.Mapping Mode"=w333:u8)  [unwired: 2 in, 2 out]
                      n193 = call "CisData.vi"("Action"=T3."Read Array", "Array No."=u32 1 ("Action")) -> ("Array OUT"=w327:dbl[])  [unwired: 3 in, 1 out]
                      n194 = property on="Cgraph" class="WFGraph (strict)"("YScale.Minimum"=w333) -> ()  [unwired: 2 in, 2 out]
                      n195 = Array Subset(array=w327, index=0, length=w336) -> (w334:dbl[])
                      n196 = Absolute Value(x=w334) -> (abs(x)=w332:dbl[])
                      n197 = case shown="..\"1/C^2 [1/nF^2]\"" w331 {
                        tunnel: [w342 w345 w348] -> w330
                        tunnel: w332 -> [w340 w347 w348]
                        frame .."1/C^2 [1/nF^2]" {
                          n198 = Array Size(array=w340) -> (size(s)=w341:i32)
                          n199 = for {
                            N: w341 -> [_]
                            tunnel: w340 -> [w344] mode=indexing
                            tunnel: [w343] -> w342 mode=indexing
                            n200 = formula code="y=1000000./(x*x);"("x"=w344) -> ("y"=w343:dbl)
                          }
                        }
                        frame "nF" {
                          n201 = Divide(x=w347, y=1000.0) -> (x/y=w345:dbl[])
                        }
                        frame "pF".. {
                        }
                      }
                      n202 = local read "Initial volts [V]"() -> (w337:dbl)
                      n203 = Bundle("Initial volts [V]"=w337, w338, w330) -> (w335:cluster{"Initial volts [V]":dbl, dbl, dbl[]})  [unwired: 1 in]
                      n204 = local write "Cgraph"(w335) -> ()
                    }
                  }
                  n205 = case shown="True" w317 {
                    tunnel: w316 -> [_ w351]
                    frame False {
                    }
                    frame True {
                      n206 = case shown="\"Log - log\".." w351 {
                        tunnel: [w352 1 0 w357] -> w350
                        tunnel: [w352 0 1 w357] -> w349
                        frame .."Lin - Lin" {
                          w352 = 0
                        }
                        frame "Log - Lin" {
                        }
                        frame "Lin - Log" {
                        }
                        frame "Log - log".. {
                          w357 = 1
                        }
                      }
                      n207 = property on="Cgraph" class="WFGraph (strict)"("X Scale.Mapping Mode"=w350) -> ()  [unwired: 2 in, 2 out]
                      n208 = property on="Cgraph" class="WFGraph (strict)"("Y Scale.Mapping Mode"=w349, "YScale.Minimum"=w349) -> ()  [unwired: 2 in, 2 out]
                    }
                  }
                  n209 = Not(x=w319) -> (.not. x?=w325:bool)
                  n210 = Greater Than 0?(x=w302) -> (x > 0?=w304:bool)
                  n211 = Format Into String(format string="%d", w302) -> (resulting string=w324:string)  [unwired: 2 in, 1 out]
                  n212 = And(x=w304, y=w325) -> (x .and. y?=w322:bool)
                  n213 = Concatenate Strings(w308, "\r\n", "Timer status: ", w324) -> (w318:string)
                  n214 = local write "STATUS 1"(w318) -> ()
                }
              }
              frame #1 {
                n215 = local read "abort"() -> (w359:bool)
                n216 = case shown="False" w359 {
                  tunnel: [w370 w518] -> w360
                  tunnel: w361 -> [w369 _]
                  tunnel: w362 -> [w368 _]
                  tunnel: [w366 w518] -> w363
                  tunnel: w364 -> [w367 _]
                  tunnel: [w365 w518] -> w358
                  frame False {
                    n217 = stacked-sequence {
                      seq-local: [w396 _ _] -> [_ w420 _]
                      seq-local: [w395 _ _] -> [_ _ w487]
                      seq-local: [w382 _ _] -> [_ _ w488]
                      tunnel: w367 -> [_ w432 w493]
                      tunnel: w368 -> [_ _ w484]
                      tunnel: [_ _ w491] -> w370
                      tunnel: [_ _ w490] -> w366
                      tunnel: w369 -> [_ _ _]
                      tunnel: [w398 _ _] -> w365
                      frame #0 {
                        w378 = T3."Write Element" ("Action")
                        # "SMU data"
                        n218 = Get Date/Time String(want seconds? (F)=TRUE) -> (time string=w397:string)  [unwired: 2 in, 1 out]
                        n219 = local write "Last reading at:"(w397) -> ()
                        n220 = local write "STATUS 1"("Reading LCR meter..." ("status")) -> ()
                        n221 = global read "QC_MeasurementSetup.vi" "Cis Measurement Parameters"() -> (w394:T8)
                        n222 = Unbundle By Name(w394) -> ("Temperature Readout"=w372:enum16{"Read Arduino", "Enter manually"}, "Arduino"=w371:refnum<class "ArduinoControl.lvclass">, "LCR"=w388:refnum<class "LCRControl.lvclass">, "AC frequency [Hz]"=w373:i32, "Supply"=w389:refnum<class "SupplyControl.lvclass">, "Set Current Limit?"=w393:bool, "Current Limit [µA]"=w391:dbl)
                        n223 = local read "Current reading No."() -> (w377:u32)
                        n224 = case shown="\"Read Arduino\"" w372 {
                          tunnel: [w405 w408] -> w375
                          tunnel: [w402 w411] -> w380
                          tunnel: w371 -> [_ w410]
                          frame "Enter manually", Default {
                            n225 = local read "Temp."() -> (w407:dbl[])
                            n226 = local read "RH"() -> (w403:dbl[])
                            n227 = Index Array(array=w407, index=0) -> (element=w405:dbl)
                            n228 = Index Array(array=w403, index=0) -> (element=w402:dbl)
                          }
                          frame "Read Arduino" {
                            n229 = call "ArduinoRead.vi"("Arduino function"=enum16{"T/RH", "Interlock", "Edgesense"}."T/RH", "ArduinoControl in"=w410) -> ("rel. Humidity [%]"=w411:dbl, "Temperature [°C]"=w408:dbl)  [unwired: 4 in, 4 out]
                          }
                        }
                        n230 = local read "Current Volts:"() -> (w381:dbl)
                        n231 = Multiply(x=w391, y=1000.0) -> (x*y=w390:dbl)
                        n232 = call-dynamic "Supply_ReadCurrent.vi"("SupplyControl in"=w389) -> ("error out"=w383:errorcluster, "Current in nA"=w399:dbl, "SupplyControl out"=w395:refnum<class "SupplyControl.lvclass">)  [unwired: 8 in]
                        n233 = case shown="True" w393 {
                          tunnel: w399 -> [_ w416]
                          tunnel: w390 -> [_ w414]
                          tunnel: [FALSE w413] -> w398
                          frame False {
                          }
                          frame True {
                            n234 = Absolute Value(x=w416) -> (abs(x)=w415:dbl)
                            n235 = Greater?(x=w415, y=w414) -> (0:w413:bool)
                          }
                        }
                        n236 = call "CisData.vi"("Action"=w378, "Array No."=0, "Array Size / Index"=w377, "Data IN"=w381) -> ()  [unwired: 1 in, 2 out]
                        n237 = call-dynamic "LCR_Readout.vi"("error in (no error)"=w383, "Frequency in Hz"=w373, "LCRControl in"=w388) -> ("error out"=w382:errorcluster, "Resistance in Ohm"=w376:dbl, "Capacitance in pF"=w374:dbl)  [unwired: 5 in, 1 out]
                        n238 = Increment(x=w377) -> (x+1=w396:u32)
                        n239 = local write "Current reading No."(w396) -> ()
                        n240 = call "CisData.vi"("Action"=w378, "Array No."=u32 1, "Array Size / Index"=w377, "Data IN"=w374) -> ()  [unwired: 1 in, 2 out]
                        n241 = call "CisData.vi"("Action"=w378, "Array No."=u32 2, "Array Size / Index"=w377, "Data IN"=w376) -> ()  [unwired: 1 in, 2 out]
                        n242 = call "CisData.vi"("Action"=w378, "Array No."=u32 3, "Array Size / Index"=w377, "Data IN"=w375) -> ()  [unwired: 1 in, 2 out]
                        n243 = call "CisData.vi"("Action"=w378, "Array No."=u32 4, "Array Size / Index"=w377, "Data IN"=w380) -> ()  [unwired: 1 in, 2 out]
                      }
                      frame #1 {
                        w429 = u32 5 ("y")
                        # "Update plots"
                        n244 = property on="Cgraph" class="WFGraph (strict)"() -> ("YScale.Mapping Mode"=w421:u8)  [unwired: 2 in, 2 out]
                        n245 = Greater?(x=w420, y=w429) -> (0:w428:bool)
                        n246 = call "CisData.vi"("Action"=T3."Read Array", "Array No."=1) -> ("Array OUT"=w418:dbl[])  [unwired: 3 in, 1 out]
                        n247 = case shown="True" w428 {
                          tunnel: w420 -> [w437 w440]
                          tunnel: w429 -> [_ w439]
                          tunnel: [w437 w439] -> w427
                          tunnel: [0 w438] -> w425
                          frame False {
                          }
                          frame True {
                            n248 = Subtract(x=w440, y=w439) -> (x-y=w438:u32)
                          }
                        }
                        n249 = property on="Cgraph" class="WFGraph (strict)"("YScale.Minimum"=w421) -> ()  [unwired: 2 in, 2 out]
                        n250 = Array Subset(array=w418, index=0, length=w420) -> (w424:dbl[])
                        n251 = local read "Cscale"() -> (w430:enum16{"1/C^2 [1/nF^2]", "nF", "pF"})
                        n252 = Absolute Value(x=w424) -> (abs(x)=w423:dbl[])
                        n253 = case shown="..\"1/C^2 [1/nF^2]\"" w430 {
                          tunnel: [w473 w476 w479] -> w435
                          tunnel: w423 -> [w471 w478 w479]
                          frame .."1/C^2 [1/nF^2]" {
                            n254 = Array Size(array=w471) -> (size(s)=w472:i32)
                            n255 = for {
                              N: w472 -> [_]
                              tunnel: w471 -> [w475] mode=indexing
                              tunnel: [w474] -> w473 mode=indexing
                              n256 = formula code="y=1000000./(x*x);"("x"=w475) -> ("y"=w474:dbl)
                            }
                          }
                          frame "nF" {
                            n257 = Divide(x=w478, y=1000.0) -> (x/y=w476:dbl[])
                          }
                          frame "pF".. {
                          }
                        }
                        n258 = for {
                          N: 5 -> [_]
                          tunnel: w427 -> [w446]
                          tunnel: w425 -> [w445]
                          tunnel: w420 -> [w444]
                          i -> [w442]
                          n259 = call "CisData.vi"("Action"=T3."Read Array", "Array No."=w442) -> ("Array OUT"=w441:dbl[])  [unwired: 3 in, 1 out]
                          n260 = case shown="2" w442 {
                            tunnel: w446 -> [w449 w453 w458 _ _]
                            tunnel: w445 -> [w450 w454 w459 _ _]
                            tunnel: w441 -> [w448 w452 w460 w464 w469]
                            tunnel: w444 -> [_ _ _ w462 w467]
                            frame ..0 {
                              n261 = Array Subset(array=w448, index=w450, length=w449) -> (w447:dbl[])
                              n262 = local write "Volts"(w447) -> ()
                            }
                            frame 1 {
                              n263 = Array Subset(array=w452, index=w454, length=w453) -> (w451:dbl[])
                              n264 = local write "Capacitance"(w451) -> ()
                            }
                            frame 2 {
                              n265 = Array Subset(array=w460, index=w459, length=w458) -> (w456:dbl[])
                              n266 = Multiply(x=w456, y=0.001) -> (x*y=w455:dbl[])
                              n267 = local write "Resistance"(w455) -> ()
                            }
                            frame 3 {
                              n268 = Decrement(x=w462) -> (x-1=w461:u32)
                              n269 = Array Subset(array=w464, index=w461, length=1) -> (w463:dbl[])
                              n270 = local write "Temp."(w463) -> ()
                            }
                            frame 4.. {
                              n271 = Decrement(x=w467) -> (x-1=w466:u32)
                              n272 = Array Subset(array=w469, index=w466, length=1) -> (w468:dbl[])
                              n273 = local write "RH"(w468) -> ()
                            }
                          }
                        }
                        n274 = local read "Initial volts [V]"() -> (w433:dbl)
                        n275 = Absolute Value(x=w432) -> (abs(x)=w431:dbl)
                        n276 = Bundle("Initial volts [V]"=w433, w431, w435) -> (w422:cluster{"Initial volts [V]":dbl, dbl, dbl[]})  [unwired: 1 in]
                        n277 = local write "Cgraph"(w422) -> ()
                      }
                      frame #2 {
                        # "Increment volts and check for end of loop"
                        n278 = local read "positive ramp?"() -> (w489:bool)
                        n279 = local read "Current Volts:"() -> (w485:dbl)
                        n280 = case shown="True" w489 {
                          tunnel: w484 -> [w496 w500]
                          tunnel: w493 -> [w497 w503]
                          tunnel: [w495 w502] -> w480
                          tunnel: [w494 w499] -> w492
                          tunnel: w485 -> [w498 w501]
                          frame False {
                            n281 = Subtract(x=w498, y=w497) -> (x-y=w494:dbl)
                            n282 = Greater Or Equal?(x=w494, y=w496) -> (x >= y?=w495:bool)
                          }
                          frame True {
                            n283 = Add(x=w501, y=w503) -> (x+y=w499:dbl)
                            n284 = Less Or Equal?(x=w499, y=w500) -> (x <= y?=w502:bool)
                          }
                        }
                        n285 = Quotient & Remainder(x=w485, y=w484) -> (x-y*floor(x/y)=w486:dbl, floor(x/y)=w483:dbl)
                        n286 = Not Equal To 0?(x=w486) -> (x != 0?=w481:bool)
                        n287 = Equal To 0?(x=w483) -> (x = 0?=w482:bool)
                        n288 = Or(x=w481, y=w482) -> ()  [unwired: 1 out]
                        n289 = case shown="True" w480 {
                          tunnel: w492 -> [_ w514]
                          tunnel: [TRUE FALSE] -> w491
                          tunnel: [FALSE w515] -> w490
                          tunnel: w485 -> [_ w512]
                          tunnel: w488 -> [_ w511]
                          tunnel: w487 -> [_ w510]
                          frame False {
                          }
                          frame True {
                            n290 = local read "step [V]"() -> (w508:dbl)
                            n291 = call "SupplyRamp.vi"("error in"=w511, "Requested Voltage"=w514, "Step Size"=w508, "Step Delay"=100, "Supply IN"=w510, "Starting Voltage"=w512) -> ("error out"=w506:errorcluster, "Compliance exceeded"=w515:bool, "Current Voltage"=w509:dbl)  [unwired: 2 in, 1 out]
                            n292 = case shown="No Error" w506 {
                              tunnel: w509 -> [w517 _]
                              frame No Error {
                                n293 = local write "Current Volts:"(w517) -> ()
                              }
                              frame Error {
                              }
                            }
                            n294 = property on="Bias On/Off:" class="Bool (strict)"("Blinking"=w515) -> ()  [unwired: 2 in, 2 out]
                            n295 = local write "STATUS 1"("Incrementing volts.") -> ()
                          }
                        }
                      }
                    }
                  }
                  frame True {
                    w518 = FALSE
                  }
                }
              }
            }
            n296 = case shown="True" w276 {
              frame False {
              }
              frame True {
                n297 = property on="Bias On/Off:" class="Bool (strict)"("Blinking"=TRUE) -> ()  [unwired: 2 in, 2 out]
              }
            }
            n298 = Build Array(w278, w276, "abort", w277) -> (w282:bool[])
            n299 = Or Array Elements(Boolean array=w282) -> (logical OR=w288:bool)
            n300 = Not(x=w288) -> (.not. x?=w287:bool)
          }
        }
        frame True {
          w520 = FALSE
          # "compliance was exceeded when first voltage applied."
          # "Flag compliance as reason for end of run"
          n301 = local write "STATUS 1"("Run aborted - compliance exceeded.") -> ()
          n302 = Build Array(w520, TRUE, w520, w520) -> (w521:bool[])
        }
      }
      n303 = Search 1D Array(1D array=w265, element=TRUE) -> (index of element=w263:i32)  [unwired: 1 in]
      n304 = Increment(x=w263) -> (x+1=w262:i32)
      n305 = case shown="..0" w262 {
        tunnel: ["" "Run ended normally" "Compliance exceeded" "Run aborted - by user" "Run aborted - Ilimit exceeded"] -> w257
        frame ..0 {
        }
        frame 1 {
        }
        frame 2 {
          # "Determine reason for end of run."
        }
        frame 3 {
        }
        frame 4.. {
        }
      }
      n306 = global read "QC_RunInformation.vi" "Run info"() -> (w261:T7)
      n307 = Bundle By Name(cluster=w261, "End of Run comment:"=w257) -> (w256:T7)
      n308 = Concatenate Strings(w257, "\r\n", "RAMPING DOWN VOLTS") -> (w260:string)
      n309 = global write "QC_RunInformation.vi" "Run info"(w256) -> ()
      n310 = local write "STATUS 1"(w260) -> ()
    }
    frame #4 {
      # "Ramp down and switch off supply"
      n311 = stacked-sequence {
        frame #0 {
          # "Tie up loose ends. Set volts to zero and switch to standby"
          # "Ramp down volts now"
          n312 = global read "QC_MeasurementSetup.vi" "Cis Measurement Parameters"() -> (w532:T8)
          n313 = Unbundle By Name(w532) -> ("Supply"=w529:refnum<class "SupplyControl.lvclass">, "Ramp down steps [V]"=w531:dbl, "Ramp down Interval [s]"=w530:i32, "Measurement switch"=w525:refnum<class "Switching.lvclass">, "Measurement switch used?"=w526:bool)
          n314 = local read "Current Volts:"() -> (w537:dbl)
          n315 = Multiply(x=w530, y=1000) -> (x*y=w534:i32)
          n316 = call "SupplyRamp.vi"("Requested Voltage"=0.0, "Step Size"=w531, "Step Delay"=w534, "Supply IN"=w529, "Starting Voltage"=w537) -> ("error out"=w528:errorcluster, "Supply OUT"=w527:refnum<class "SupplyControl.lvclass">, "Current Voltage"=w535:dbl)  [unwired: 3 in, 1 out]
          n317 = call-dynamic "Supply_Stby.vi"("error in (no error)"=w528, "SupplyControl in"=w527) -> ("error out"=w524:errorcluster)  [unwired: 8 in, 1 out]
          n318 = local write "Current Volts:"(w535) -> ()
          n319 = case shown="True" w526 {
            tunnel: w525 -> [_ w540]
            tunnel: w524 -> [_ w538]
            frame False {
            }
            frame True {
              n320 = call-dynamic "MatrixSwitch.vi"("error in (no error)"=w538, "Action"=T4."Reset", "Switching in"=w540) -> ()  [unwired: 6 in, 3 out]
            }
          }
        }
        frame #1 {
          w545 = 0
          n321 = local write "Bias On/Off:"(FALSE ("Visible")) -> ()
          n322 = local write "Current Volts:"(0.0 ("Current Volts:")) -> ()
          n323 = property on="abort" class="Bool (strict)"("DisabledEnum"=2) -> ()  [unwired: 2 in, 2 out]
          n324 = property on="Quit & Save" class="Bool"("DisabledEnum"=w545) -> ()  [unwired: 2 in, 2 out]
          n325 = property on="quit (no save)" class="Bool"("DisabledEnum"=w545) -> ()  [unwired: 2 in, 2 out]
          n326 = local write "STATUS 1"("Run finished. \nSave data?" ("STATUS 1")) -> ()
        }
        frame #2 {
          n327 = Current VI's Path() -> (path=w547:path)
          n328 = call "SaveJPEG.vi"("Test"="Cis", "File Path Control"=w547) -> ()  [unwired: 1 in, 2 out]
        }
      }
    }
    frame #5 {
      # "Loop and await decision on whether to save or junk data"
      # "Display and save data"
      n329 = local read "Cscale"() -> (w558:enum16{"1/C^2 [1/nF^2]", "nF", "pF"})
      n330 = local read "Scales"() -> (w559:T1)
      n331 = while {
        shift-left: w558 -> [w609]
        shift-right: [w608] -> _
        shift-left: w559 -> [w611]
        shift-right: [w610] -> _
        tunnel: ["Quit & Save"] -> w561
        tunnel: ["quit (no save)"] -> w560
        stop <- w606 continue-if-true
        n332 = local read "Scales"() -> (w610:T1)
        n333 = local read "Cscale"() -> (w608:enum16{"1/C^2 [1/nF^2]", "nF", "pF"})
        n334 = Not Equal?(x=w611, y=w610) -> (x != y?=w604:bool)
        n335 = Not Equal?(x=w609, y=w608) -> (x != y?=w603:bool)
        n336 = case shown="True" w604 {
          tunnel: w610 -> [_ w638]
          frame False {
          }
          frame True {
            n337 = case shown="\"Log - log\".." w638 {
              tunnel: [w639 1 0 w644] -> w637
              tunnel: [w639 0 1 w644] -> w636
              frame .."Lin - Lin" {
                w639 = 0
              }
              frame "Log - Lin" {
              }
              frame "Lin - Log" {
              }
              frame "Log - log".. {
                w644 = 1
              }
            }
            n338 = property on="Cgraph" class="WFGraph (strict)"("X Scale.Mapping Mode"=w637) -> ()  [unwired: 2 in, 2 out]
            n339 = property on="Cgraph" class="WFGraph (strict)"("Y Scale.Mapping Mode"=w636, "YScale.Minimum"=w636) -> ()  [unwired: 2 in, 2 out]
          }
        }
        n340 = case shown="True" w603 {
          tunnel: w608 -> [_ w616]
          frame False {
          }
          frame True {
            n341 = property on="Cgraph" class="WFGraph (strict)"() -> ("YScale.Mapping Mode"=w619:u8)  [unwired: 2 in, 2 out]
            n342 = global read "QC_MeasurementSetup.vi" "Cis Measurement Parameters"() -> (w618:T8)
            n343 = property on="Cgraph" class="WFGraph (strict)"("YScale.Minimum"=w619) -> ()  [unwired: 2 in, 2 out]
            n344 = Unbundle By Name(w618) -> ("Initial Voltage [V]"=w621:dbl, "Step Size [V]"=w623:dbl, "Number Of Steps"=w620:u32)
            n345 = call "CisData.vi"("Action"=T3."Read Array", "Array No."=u32 1 ("Action")) -> ("Array OUT"=w612:dbl[])  [unwired: 3 in, 1 out]
            n346 = Absolute Value(x=w623) -> (abs(x)=w622:dbl)
            n347 = Array Subset(array=w612, index=0, length=w620) -> (w624:dbl[])
            n348 = Absolute Value(x=w624) -> (abs(x)=w617:dbl[])
            n349 = case shown="..\"1/C^2 [1/nF^2]\"" w616 {
              tunnel: [w629 w632 w635] -> w615
              tunnel: w617 -> [w627 w634 w635]
              frame .."1/C^2 [1/nF^2]" {
                n350 = Array Size(array=w627) -> (size(s)=w628:i32)
                n351 = for {
                  N: w628 -> [_]
                  tunnel: w627 -> [w631] mode=indexing
                  tunnel: [w630] -> w629 mode=indexing
                  n352 = formula code="y=1000000./(x*x);"("x"=w631) -> ("y"=w630:dbl)
                }
              }
              frame "nF" {
                n353 = Divide(x=w634, y=1000.0) -> (x/y=w632:dbl[])
              }
              frame "pF".. {
              }
            }
            n354 = Bundle("Initial Voltage [V]"=w621, w622, w615) -> (w625:cluster{"Initial Voltage [V]":dbl, dbl, dbl[]})  [unwired: 1 in]
            n355 = local write "Cgraph"(w625) -> ()
          }
        }
        n356 = local read "Run uninterrupted?"() -> (w602:bool)
        n357 = Compound Arithmetic op=OR("Quit & Save", "quit (no save)", w602) -> (invert w606:bool)
      }
      n358 = global read "QC_MeasurementSetup.vi" "Cis Measurement Parameters"() -> (w557:T8)
      n359 = Unbundle By Name(w557) -> ("Temperature Readout"=w556:enum16{"Read Arduino", "Enter manually"}, "Arduino"=w550:refnum<class "ArduinoControl.lvclass">)
      n360 = case shown="\"Read Arduino\"" w556 {
        tunnel: w550 -> [_ w601]
        frame "Enter manually", Default {
        }
        frame "Read Arduino" {
          n361 = call "ArduinoClose.vi"("ArduinoControl in"=w601) -> ()  [unwired: 9 in, 2 out]
        }
      }
      n362 = case shown="True" w560 {
        tunnel: [FALSE w646] -> w562
        frame False {
        }
        frame True {
          n363 = Two Button Dialog(message="Are you sure you don't want to save the data?", 1:"Quit" ("F button name (\"Cancel\")"), 2:"Save data" ("T button name (\"OK\")")) -> (T button?=w646:bool)
        }
      }
      n364 = local read "Run uninterrupted?"() -> (w548:bool)
      n365 = Compound Arithmetic op=OR(w561, w562, w548) -> (w555:bool)
      n366 = flat-sequence {
        tunnel: w555 -> [w565]
        tunnel: [w565] -> w551
        tunnel: [TRUE] -> w549
        tunnel: w548 -> [w563]
        frame #0 {
          n367 = case shown="True" w565 {
            tunnel: ["" w600] -> w575
            tunnel: [_ w585] -> w573
            tunnel: w563 -> [_ w578]
            frame False {
            }
            frame True {
              w583 = T3."Read Array" ("Action")
              n368 = local write "STATUS 1"("Saving Data ...") -> ()
              n369 = call "CisData.vi"("Action"=w583, "Array No."=u32 2 ("Action")) -> ("Array OUT"=w581:dbl[])  [unwired: 3 in, 1 out]
              n370 = call "CisData.vi"("Action"=w583, "Array No."=u32 4 ("Action")) -> ("Array OUT"=w597:dbl[])  [unwired: 3 in, 1 out]
              n371 = call "CisData.vi"("Action"=w583, "Array No."=u32 3 ("Action")) -> ("Array OUT"=w596:dbl[])  [unwired: 3 in, 1 out]
              n372 = call <vilib>:"Std Deviation and Variance.vi"("X"=w597) -> ("mean"=w586:dbl)  [unwired: 1 in, 2 out]
              n373 = call <vilib>:"Std Deviation and Variance.vi"("X"=w596) -> ("mean"=w587:dbl)  [unwired: 1 in, 2 out]
              n374 = Multiply(x=w581, y=0.001) -> (x*y=w580:dbl[])
              n375 = call "CisData.vi"("Action"=w583, "Array No."=u32 0 ("Action")) -> ("Array OUT"=w591:dbl[])  [unwired: 3 in, 1 out]
              n376 = call "CisData.vi"("Action"=w583, "Array No."=u32 1 ("Action")) -> ("Array OUT"=w590:dbl[])  [unwired: 3 in, 1 out]
              n377 = Build Array(w591, w590, w580) -> (w589:dbl[][])
              n378 = Transpose 2D Array(2D array=w589) -> (transposed array=w577:dbl[][])
              n379 = call "SaveDataFile.vi"("Data Array"=w577, "Temperature"=w587, "Run uninterrupted?"=w578, "Humidity"=w586, "Array Titles"="Voltage[V] Capacitance[pF] Resistance[kOhm]", "Strip Segment"="", "Arrays format"="%010.2f") -> ("Path + Filename OUT"=w600:string, "Error Out"=w585:errorcluster)  [unwired: 5 in, 2 out]
            }
          }
          n380 = global read "QC_MeasurementSetup.vi" "Cis Measurement Parameters"() -> (w574:T8)
          n381 = Unbundle By Name(w574) -> ("C_is Limit [pF/cm]"=w568:dbl)
          n382 = call "ScanFeedback.vi"("measurement type"=T5."Cis") -> ("Cis @300V [pF/cm]"=w566:dbl)  [unwired: 4 in, 4 out]
          n383 = Absolute Value(x=w566) -> (abs(x)=w569:dbl)
          n384 = Absolute Value(x=w568) -> (abs(x)=w567:dbl)
          n385 = Less Or Equal?(x=w569, y=w567) -> (x <= y?=w570:bool)
          n386 = call "WriteLogFile.vi"("Run uninterrupted?"=w563, "Automatic warning"="", "Data File"=w575, "Error In"=w573, "DUT passed?"=w570, "Value TechSpec criteria"=w566, "Files saved?"=w565) -> ()  [unwired: 4 in, 1 out]
        }
      }
      n387 = Select(t="Run finished.\nData saved." ("STATUS 1"), s=w551, f="Run finished.\nData not saved." ("STATUS 1")) -> (s? t:f=w554:string)
      n388 = local write "STATUS 1"(w554) -> ()
      "Done!" <- w549
    }
  }
